vi "build_component_classpath.vi"(1 "1st_level_parent (in)":refnum<k20>, 2 "comp_name (in)":string, 5 "error in (no error)":errorcluster) -> (16 "classpath (out)":string, 19 "error out":errorcluster)   [LabVIEW 2016]
uses:
  <vilib>/xml/Close Reference(Node).vi
  <resource>/objmgr/DOMUserDefRef.rc
  <vilib>/xml/NI_XML.lvlib
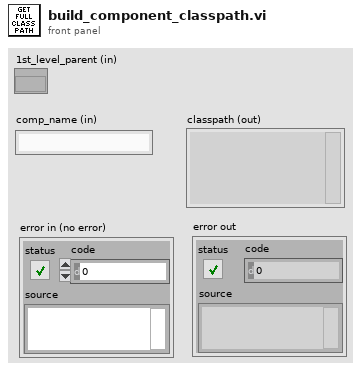
[diagram p1: front panel]
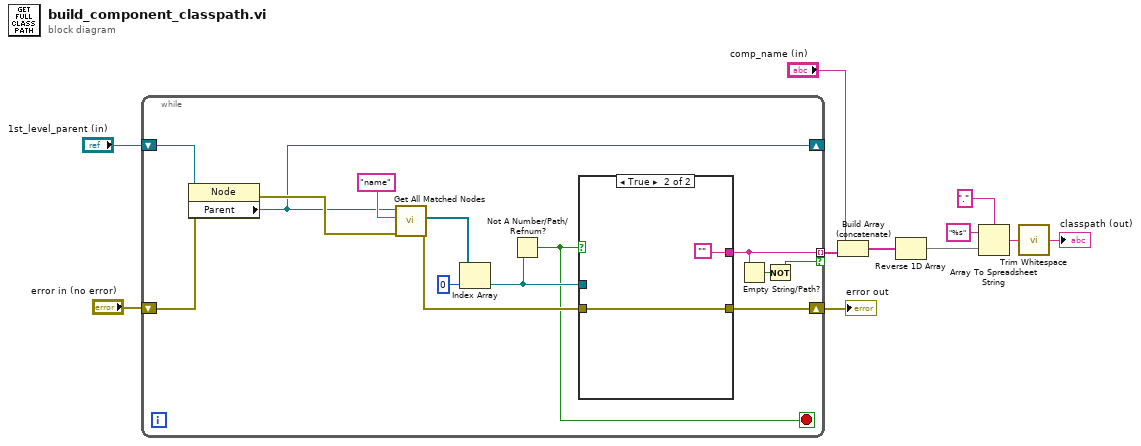
[diagram p0: block diagram]
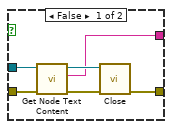
[diagram p2: hidden frame]
diagram:
  n1 = while {
    shift-right: [w19] -> _
    shift-left: "1st_level_parent (in)" -> [w20]
    shift-right: [w16] -> w9
    shift-left: "error in (no error)" -> [w17]
    tunnel: [w14] -> w8 mode=indexing if=w12
    stop <- w15 stop-if-true
    n2 = property class="Node"(reference=w20, error in=w17) -> (error out=w23:errorcluster, "Parent"=w19:refnum<k20>)  [unwired: 1 out]
    n3 = call <vilib>:"Get All Matched Nodes.vi"("error in (no error)"=w23, "XPath expression"="name", "node in"=w19) -> ("error out"=w21:errorcluster, "node result array"=w22:refnum<k20>[])  [unwired: 6 in, 1 out]
    n4 = Index Array(array=w22, index=0) -> (element=w18:refnum<k20>)
    n5 = Not A Number/Path/Refnum?(number/path/refnum=w18) -> (NaN/Path/Refnum?=w15:bool)
    n6 = case shown="True" w15 {
      tunnel: w21 -> [w31 w33]
      tunnel: w18 -> [w30 _]
      tunnel: [w27 w33] -> w16
      tunnel: [w26 ""] -> w14
      frame False {
        n7 = call <vilib>:"Get Node Text Content.vi"("error in (no error)"=w31, "node in"=w30) -> ("error out"=w28:errorcluster, "node text"=w26:string, "node out"=w29:refnum<k20>)  [unwired: 7 in]
        n8 = call-poly <vilib>:"Close.vi"("error in (no error)"=w28, "node"=w29) -> ("error out"=w27:errorcluster)  [unwired: 7 in]
      }
      frame True {
      }
    }
    n9 = Empty String/Path?(string/path=w14) -> (empty?=w13:bool)
    n10 = Not(x=w13) -> (.not. x?=w12:bool)
  }
  "error out" <- w9
  n11 = Build Array (concatenate)("comp_name (in)", w8) -> (w6:string[])
  n12 = Reverse 1D Array(array=w6) -> (reversed array=w1:string[])
  n13 = Array To Spreadsheet String(delimiter (Tab)=".", array=w1, 3:"%s" ("format string")) -> (spreadsheet string=w3:string)
  n14 = call <vilib>:"Trim Whitespace.vi"("string"=w3) -> ("trimmed string"=→"classpath (out)":string)  [unwired: 1 in]
